vi "例4.3-1 比较大小（条件结构）.vi"() -> ()   [LabVIEW 2017]
panel:
  out "max":dbl
  in  "b":dbl
  in  "a":dbl
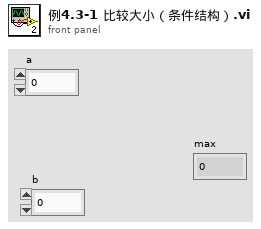
[diagram p1: front panel]
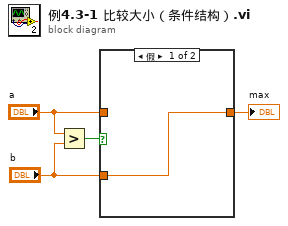
[diagram p0: block diagram]
diagram:
  n1 = Greater?(x="a", y="b") -> (0:w4:bool)
  n2 = case shown="假" w4 {
    tunnel: "a" -> [_ w6]
    tunnel: [w5 w6] -> w2
    tunnel: "b" -> [w5 _]
    frame False {
    }
    frame True {
    }
  }
  "max" <- w2
